vi "Test RFP_Flash_once.bat.vi"(8 "error in (no error)":errorcluster, 9 "Project":string="k7000_2.rpj", 10 "RFP Auto Path":string=".\\RFP_Auto\\Scripts\\Flash_once.bat", 11 "SN":string="ABCSN") -> (0 "error out":errorcluster, 2 "RFP Log Path":string, 3 "Result":bool)   [LabVIEW 2024]
panel:
  out "path":path=path "D:/WeiFu/Labview ATS/Customer_Zhuo/RF_Download/ATS/Project/RFP_Auto/Scripts/Flash_once.bat"
  out "original":string="@echo off\nsetlocal enabledelayedexpansion\n\nREM ========= 用户可配置区 =========\nset RFP_DIR=C:\\Program Files (x86)\\Renesas Electronics\\Programming Tools\\Renesas Flash Programmer V3.16\nset RFP_EXE=%RFP_DIR%\\RFPV3.exe\nset RFP_CONSOLE=%RFP_DIR%\\RFPV3.Console.exe\n\nset PROJECT=D:\\Alvin\\1.Project\\5.ZhiRuiJia\\Flash\\RFP_Auto\\Project\\k7001.rpj\nREM 固件已配置在 .rpj 内，这里默认不再单独指定 /file\nset FIRMWARE=\nset LOG_DIR=D:\\Alvin\\1.Project\\5.ZhiRuiJia\\Flash\\RFP_Auto\\Logs\nset RETRY=2\nREM 可选：如果你只有一台E2 Lite，通常不需要指定tool序列号\nset TOOL_SN=\nREM 示例：set TOOL_SN=xxxxxxxxx\nREM =================================\n\nif not exist \"%LOG_DIR%\" mkdir \"%LOG_DIR%\"\n\nREM SN 可由扫码枪/上位机传入：flash_once.bat SNABCSN\nset SN=%1\nif \"%SN%\"==\"\" set SN=NO_SN\n\nREM 时间戳（yyyyMMdd_HHmmss）\nfor /f %%i in ('powershell -NoProfile -Command \"Get-Date -Format yyyyMMdd_HHmmss\"') do set TS=%%i\n\nset LOG_FILE=%LOG_DIR%\\%SN%_%TS%.log\n\necho [INFO] SN=%SN%\necho [INFO] Project=%PROJECT%\nif not \"%FIRMWARE%\"==\"\" echo [INFO] Firmware=%FIRMWARE%\necho [INFO] Log=%LOG_FILE%\necho.\n\nREM 参数拼接\nset COMMON_ARGS=/silent \"%PROJECT%\" /command epv /log \"%LOG_FILE%\"\nif not \"%FIRMWARE%\"==\"\" set COMMON_ARGS=%COMMON_ARGS% /file \"%FIRMWARE%\"\nif not \"%TOOL_SN%\"==\"\" set COMMON_ARGS=%COMMON_ARGS% /tool %TOOL_SN%\n\nset /a COUNT=0\n\n:RETRY_LOOP\nset /a COUNT+=1\necho [INFO] Attempt !COUNT! ...\n\nREM 优先用 RFPV3.exe /silent\n\"%RFP_EXE%\" %COMMON_ARGS%\nset RC=%ERRORLEVEL%\n\necho [INFO] ExitCode=%RC%\n\nif \"%RC%\"==\"0\" goto PASS\n\nif !COUNT! LEQ %RETRY% (\n    echo [WARN] Programming failed, retrying...\n    timeout /t 2 >nul\n    goto RETRY_LOOP\n)\n\ngoto FAIL\n\n:PASS\nfor /f %%i in ('powershell -NoProfile -Command \"Get-Date -Format yyyyMMdd_HHmmss\"') do set END_TS=%%i\necho [INFO] EndTime=%END_TS%\necho [PASS] %SN% %TS% >> \"%LOG_DIR%\\summary_pass.txt\"\necho SUCCESS\nexit /b 0\n\n:FAIL\nfor /f %%i in ('powershell -NoProfile -Command \"Get-Date -Format yyyyMMdd_HHmmss\"') do set END_TS=%%i\necho [INFO] EndTime=%END_TS%\necho [FAIL] %SN% %TS% ExitCode=%RC% >> \"%LOG_DIR%\\summary_fail.txt\"\necho FAIL\nexit /b 1\n"
  # "D:\\WeiFu\\Labview ATS\\Customer_Zhuo\\RF_Download\\ATS\\Project\\RFP_Auto\\Scripts\\Flash_once.bat"
  # "..\\RFP_Auto\\Scripts\\Flash_once.bat"
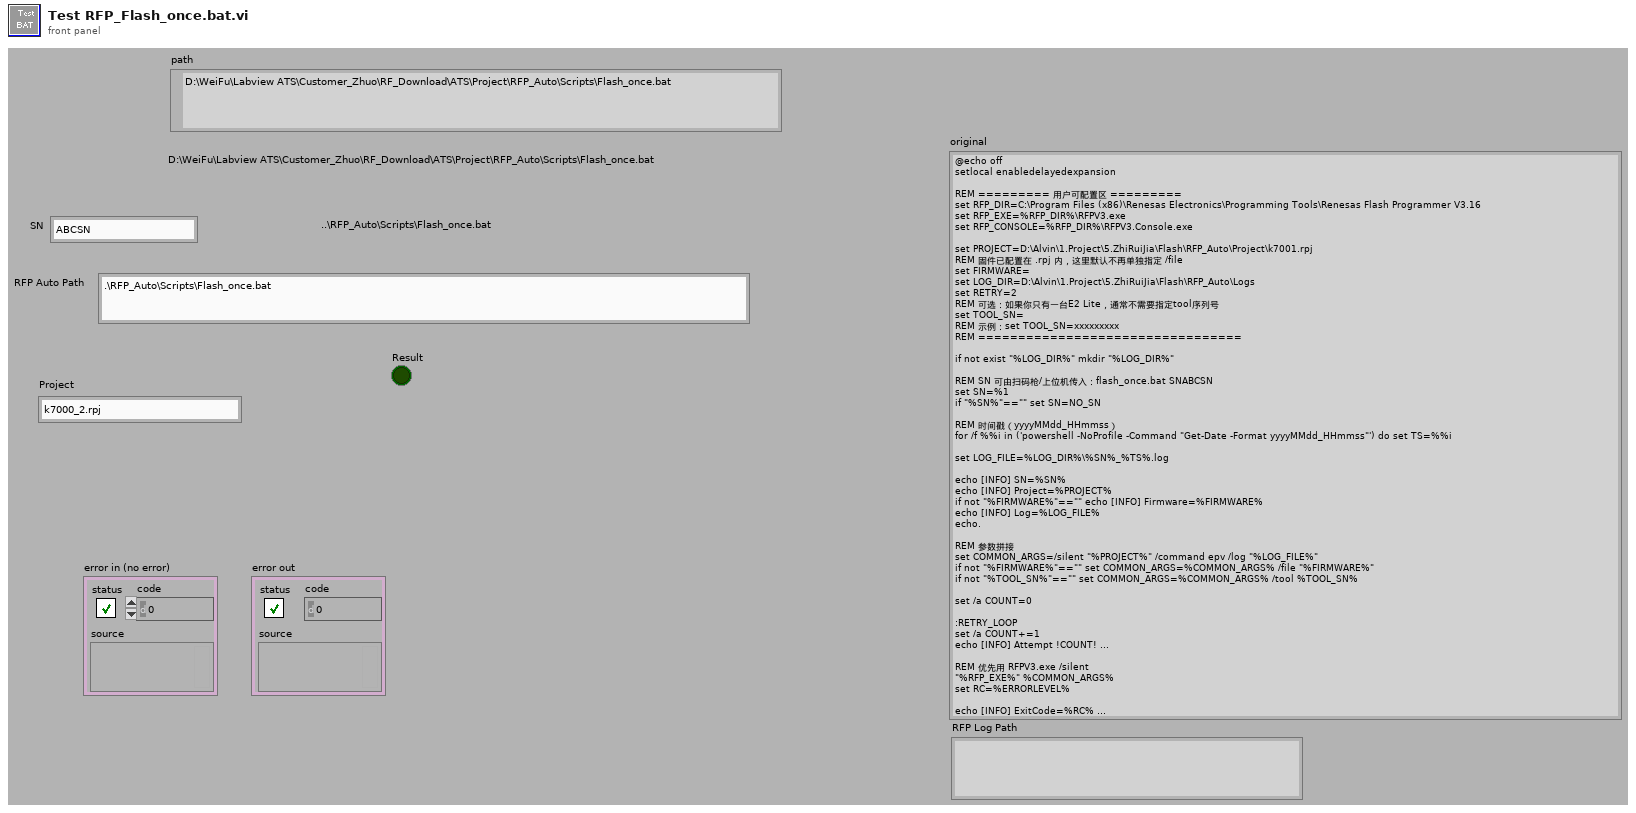
[diagram p1: front panel]
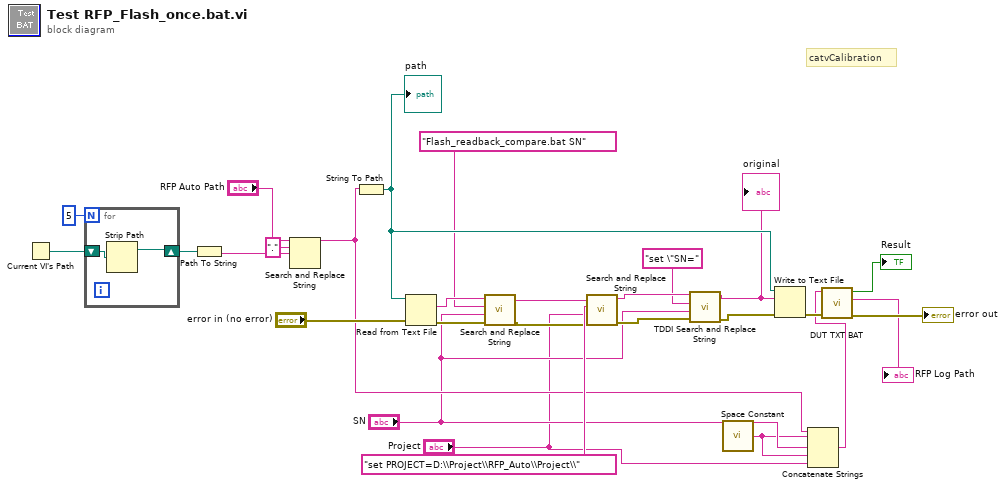
[diagram p0: block diagram]
diagram:
  # "catvCalibration"
  n1 = Current VI's Path() -> (path=w23:path)
  n2 = for {
    N: 5 -> [_]
    shift-right: [w29] -> w21
    shift-left: w23 -> [w30]
    n3 = Strip Path(path=w30) -> (stripped path=w29:path)  [unwired: 1 out]
  }
  n4 = Path To String(path=w21) -> (string=w18:string)
  n5 = Search and Replace String(input string="RFP Auto Path", search string=".", replace string=w18) -> (result string=w5:string)  [unwired: 5 in, 3 out]
  n6 = String To Path(string=w5) -> (path=w24:path)
  "path" <- w24
  n7 = Read from Text File(file (use dialog)=w24, error in="error in (no error)") -> (text=w17:string, error out=w15:errorcluster)  [unwired: 2 in, 2 out]
  n8 = call "Search and Replace String.vi"("error in (no error)"=w15, "Replace Str"="SN", "FindStr"="Flash_readback_compare.bat SN", "originalTex"=w17) -> ("error out"=w11:errorcluster, "output Str"=w12:string)  [unwired: 6 in]
  n9 = call "Search and Replace String.vi"("error in (no error)"=w11, "Replace Str"="Project", "FindStr"="set PROJECT=D:\\Project\\RFP_Auto\\Project\\", "originalTex"=w12) -> ("error out"=w10:errorcluster, "output Str"=w9:string)  [unwired: 6 in]
  n10 = call "TDDI Search and Replace String.vi"("error in (no error)"=w10, "Replace Str"="SN", "FindStr"="set \"SN=", "originalTex"=w9) -> ("error out"=w7:errorcluster, "output Str"=w8:string)  [unwired: 6 in]
  "original" <- w8
  n11 = call <vilib>:"Space Constant.vi"() -> ("String"=w3:string)
  n12 = Write to Text File(file (use dialog)=w24, text=w8, error in=w7) -> (error out=w28:errorcluster)  [unwired: 1 in, 2 out]
  n13 = Concatenate Strings(w5, w3, "SN", w3, "Project") -> (w1:string)
  n14 = call "DUT TXT BAT.vi"("error in (no error)"=w28, "command line"=w1) -> ("error out"=→"error out":errorcluster, "Log Path"=→"RFP Log Path":string, "Result"=→"Result":bool)  [unwired: 7 in]
